vi "LD TrayFGV.vi"(9 "Status":string, 10 "Insert":i32, 11 "Enum":T1) -> (2 "Array":string[](array[string]), 3 "Read":string)   [LabVIEW 2019]
uses:
  Ctrl/123.ctl
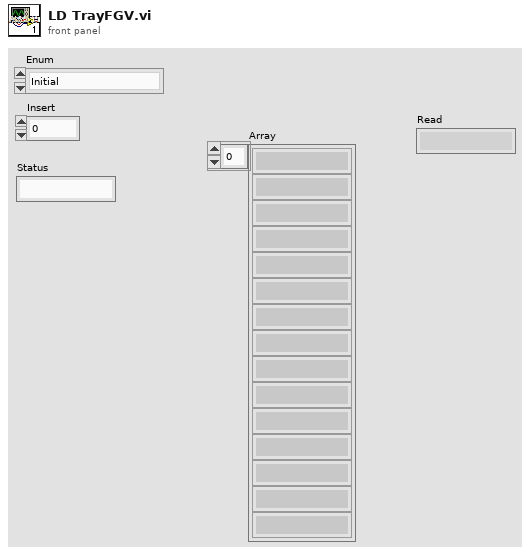
[diagram p1: front panel]
types:
  T1 = typedef "123.ctl" = enum16{"Initial", "Write", "Read"}
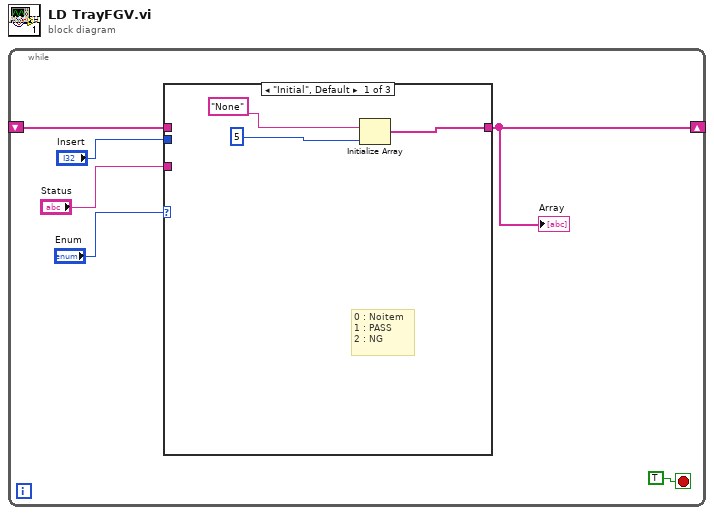
[diagram p0: block diagram]
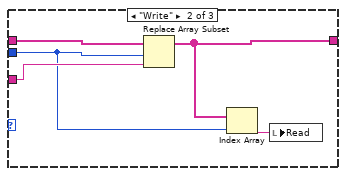
[diagram p2: hidden frame]
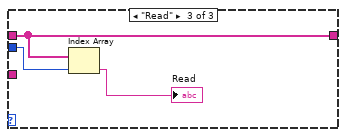
[diagram p3: hidden frame]
diagram:
  n1 = while {
    shift-right: [w1] -> _
    shift-left: _ -> [w5]
    stop <- TRUE stop-if-true
    n2 = case shown="\"Initial\", Default" "Enum" {
      tunnel: w5 -> [_ w13 w17]
      tunnel: [w8 w11 w17] -> w1
      tunnel: "Insert" -> [_ w12 w16]
      tunnel: "Status" -> [_ w14 _]
      frame "Initial", Default {
        # "0 : Noitem\n1 : PASS\n2 : NG"
        n3 = Initialize Array("None", 5 ("dimension size")) -> (w8:string[])
      }
      frame "Write" {
        n4 = Replace Array Subset "Replace Array Subset"(array=w13, new element=w14, index=w12) -> (w11:string[])
        n5 = Index Array(array=w11, index=w12) -> (element=w10:string)
        n6 = local write "Read"(w10) -> ()
      }
      frame "Read" {
        n7 = Index Array(array=w17, index=w16) -> (element=→"Read":string)
      }
    }
    "Array" <- w1
  }
